vi "Pfeiffer-RVC300.add services.vi"(0 "i ref in":refnum<vi>, 3 "ms timeout (10000)":i32=10000, 5 "error in (no error)":errorcluster) -> (14 "i ref out":refnum<vi>, 17 "timed out":bool, 19 "error out":errorcluster)   [LabVIEW 2014, in "Pfeiffer-RVC300.lvlib"]
doc: "Declares the required DIM services."
uses:
  Pfeiffer-RVC300.lvlib
  Pfeiffer-RVC300.regulation mode.ctl
  CSlibraries-extern/DimLVEvent/LVDimInterface/LVDimInterface.lvlib
  CSCore/CSSystem/CSSystemLib/CSSystemLib.lvlib
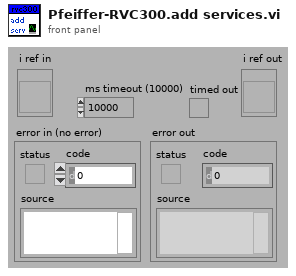
[diagram p1: front panel]
types:
  T1 = typedef "Pfeiffer-RVC300.lvlib/Pfeiffer-RVC300.i attribute.ctl" = cluster{"interfaceInitialized":bool, "VISAResource":refnum<visa-resource-name>, "WaitingTime":u32, "nomValues":T2, "actValues":T2}
  T2 = typedef "Pfeiffer-RVC300.lvlib/Pfeiffer-RVC300.parameters.ctl" = cluster{"regulationMode":T3, "valveType":string, "sensorType":string, "valveState":string, "flow":dbl, "pressure":dbl, "serviceIDs":cluster{"regulationModeID":i32, "valveTypeID":i32, "sensorTypeID":i32, "valveStateID":i32, "flowID":i32, "pressureID":i32}}
  T3 = typedef "Pfeiffer-RVC300.lvlib/Pfeiffer-RVC300.regulation mode.ctl" = enum16{"unknown", "Pressure", "Flow", "Wait"}
  T4 = cluster{"my_serviceID":i32, "my_serviceID":i32, "my_serviceID":i32, "my_serviceID":i32, "my_serviceID":i32, "my_serviceID":i32}
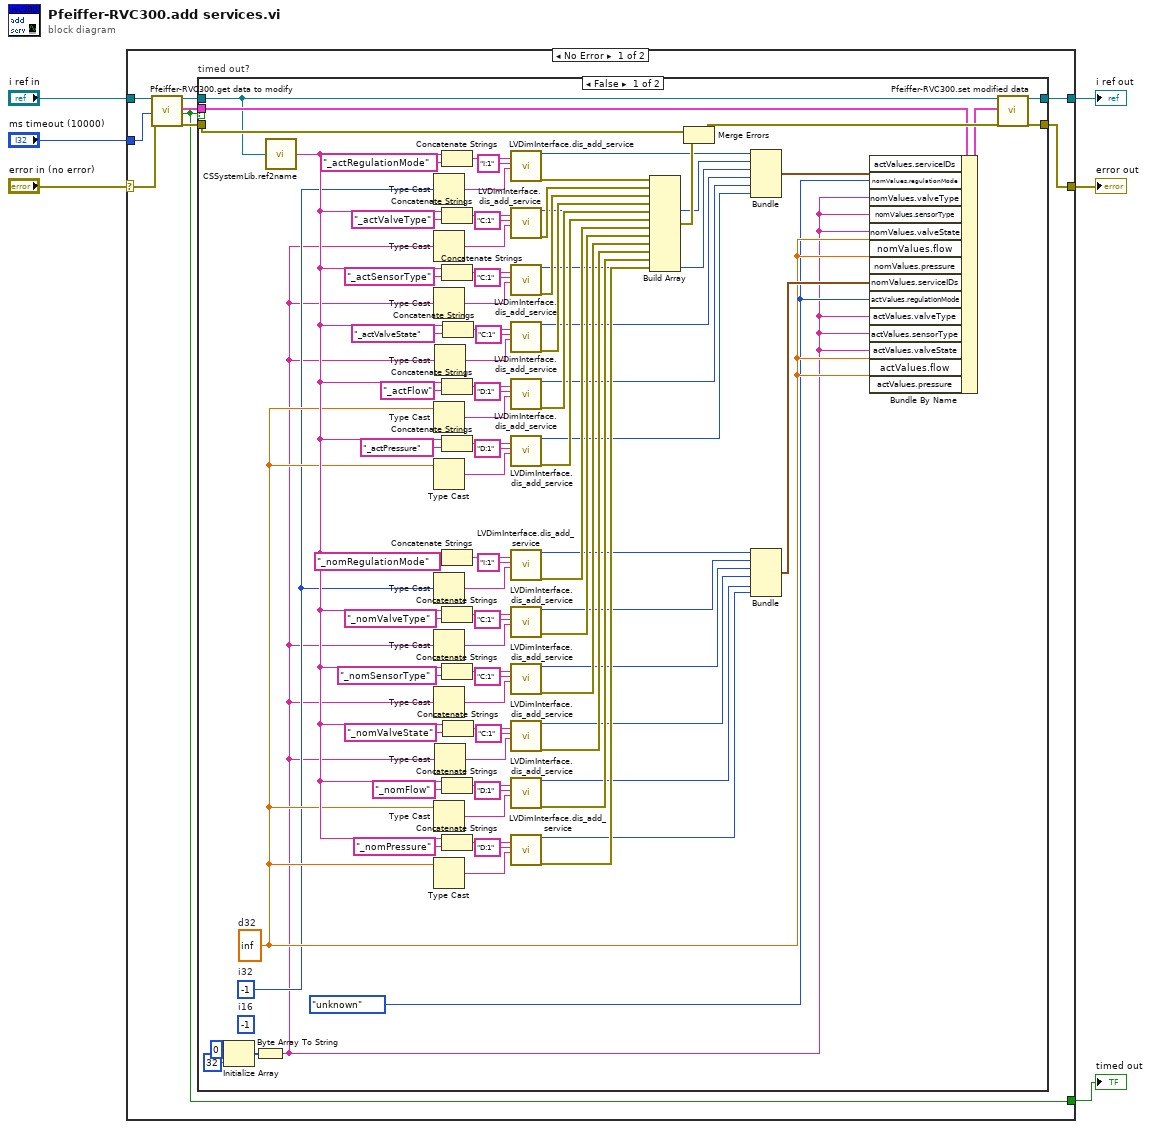
[diagram p0: block diagram]
diagram:
  n1 = case shown="No Error" "error in (no error)" {
    selector: "error in (no error)" -> [w13 w109]
    tunnel: [w9 w109] -> w5
    tunnel: "i ref in" -> [w15 w108]
    tunnel: [w11 w108] -> w3
    tunnel: "ms timeout (10000)" -> [w14 _]
    tunnel: [w8 _] -> w1
    frame No Error {
      n2 = call "Pfeiffer-RVC300.get data to modify.vi"("i ref in"=w15, "ms timeout (10000)"=w14, "error in (no error)"=w13) -> ("i ref out"=w12:refnum<vi>, "i attribute"=w7:T1, "timed out"=w8:bool, "error out"=w10:errorcluster)  [unwired: 13 in]
      n3 = case "timed out?" shown="False" w8 {
        tunnel: w12 -> [w25 w107]
        tunnel: [w105 w107] -> w11
        tunnel: w10 -> [w42 w106]
        tunnel: [w104 w106] -> w9
        tunnel: w7 -> [w39 _]
        frame False {
          w20 = Pfeiffer-RVC300.regulation_mode."unknown" ("actValues.regulationMode")
          (unwired) i16 -1  # i16
          w22 = inf  # d32
          w21 = -1  # i32
          n4 = Initialize Array(u8 0, 32 ("dimension size")) -> (w19:u8[])
          n5 = Byte Array To String(unsigned byte array=w19) -> (string=w16:string)
          n6 = call "CSSystemLib.ref2name.vi"("obj refnum"=w25) -> ("name"=w55:string)
          n7 = Type Cast(x=w21) -> (*(type *) &x=w100:string)  [unwired: 1 in]
          n8 = Type Cast(x=w16) -> (*(type *) &x=w99:string)  [unwired: 1 in]
          n9 = Type Cast(x=w16) -> (*(type *) &x=w92:string)  [unwired: 1 in]
          n10 = Type Cast(x=w22) -> (*(type *) &x=w84:string)  [unwired: 1 in]
          n11 = Type Cast(x=w22) -> (*(type *) &x=w80:string)  [unwired: 1 in]
          n12 = Type Cast(x=w21) -> (*(type *) &x=w76:string)  [unwired: 1 in]
          n13 = Type Cast(x=w16) -> (*(type *) &x=w75:string)  [unwired: 1 in]
          n14 = Type Cast(x=w16) -> (*(type *) &x=w68:string)  [unwired: 1 in]
          n15 = Type Cast(x=w22) -> (*(type *) &x=w60:string)  [unwired: 1 in]
          n16 = Type Cast(x=w22) -> (*(type *) &x=w56:string)  [unwired: 1 in]
          n17 = Type Cast(x=w16) -> (*(type *) &x=w88:string)  [unwired: 1 in]
          n18 = Type Cast(x=w16) -> (*(type *) &x=w64:string)  [unwired: 1 in]
          n19 = Concatenate Strings(w55, "_actRegulationMode" ("string")) -> (w103:string)
          n20 = Concatenate Strings(w55, "_actValveType" ("string")) -> (w96:string)
          n21 = Concatenate Strings(w55, "_actSensorType" ("string")) -> (w95:string)
          n22 = Concatenate Strings(w55, "_actFlow" ("string")) -> (w87:string)
          n23 = Concatenate Strings(w55, "_actPressure" ("string")) -> (w83:string)
          n24 = Concatenate Strings(w55, "_nomRegulationMode" ("string")) -> (w79:string)
          n25 = Concatenate Strings(w55, "_nomValveType" ("string")) -> (w72:string)
          n26 = Concatenate Strings(w55, "_nomSensorType" ("string")) -> (w71:string)
          n27 = Concatenate Strings(w55, "_nomFlow" ("string")) -> (w63:string)
          n28 = Concatenate Strings(w55, "_nomPressure" ("string")) -> (w59:string)
          n29 = Concatenate Strings(w55, "_actValveState" ("string")) -> (w91:string)
          n30 = Concatenate Strings(w55, "_nomValveState" ("string")) -> (w67:string)
          n31 = call "LVDimInterface.dis_add_service.vi"("serviceName"=w103, "typeDescriptor"="I:1", "data"=w100) -> ("my_serviceID"=w38:i32, "error out"=w54:errorcluster)  [unwired: 15 in]
          n32 = call "LVDimInterface.dis_add_service.vi"("serviceName"=w96, "typeDescriptor"="C:1", "data"=w99) -> ("my_serviceID"=w37:i32, "error out"=w53:errorcluster)  [unwired: 15 in]
          n33 = call "LVDimInterface.dis_add_service.vi"("serviceName"=w95, "typeDescriptor"="C:1", "data"=w92) -> ("my_serviceID"=w36:i32, "error out"=w52:errorcluster)  [unwired: 15 in]
          n34 = call "LVDimInterface.dis_add_service.vi"("serviceName"=w91, "typeDescriptor"="C:1", "data"=w88) -> ("my_serviceID"=w35:i32, "error out"=w51:errorcluster)  [unwired: 15 in]
          n35 = call "LVDimInterface.dis_add_service.vi"("serviceName"=w87, "typeDescriptor"="D:1", "data"=w84) -> ("my_serviceID"=w34:i32, "error out"=w50:errorcluster)  [unwired: 15 in]
          n36 = call "LVDimInterface.dis_add_service.vi"("serviceName"=w83, "typeDescriptor"="D:1", "data"=w80) -> ("my_serviceID"=w33:i32, "error out"=w49:errorcluster)  [unwired: 15 in]
          n37 = call "LVDimInterface.dis_add_service.vi"("serviceName"=w79, "typeDescriptor"="I:1", "data"=w76) -> ("my_serviceID"=w32:i32, "error out"=w48:errorcluster)  [unwired: 15 in]
          n38 = call "LVDimInterface.dis_add_service.vi"("serviceName"=w72, "typeDescriptor"="C:1", "data"=w75) -> ("my_serviceID"=w31:i32, "error out"=w47:errorcluster)  [unwired: 15 in]
          n39 = call "LVDimInterface.dis_add_service.vi"("serviceName"=w71, "typeDescriptor"="C:1", "data"=w68) -> ("my_serviceID"=w30:i32, "error out"=w46:errorcluster)  [unwired: 15 in]
          n40 = call "LVDimInterface.dis_add_service.vi"("serviceName"=w67, "typeDescriptor"="C:1", "data"=w64) -> ("my_serviceID"=w29:i32, "error out"=w45:errorcluster)  [unwired: 15 in]
          n41 = call "LVDimInterface.dis_add_service.vi"("serviceName"=w63, "typeDescriptor"="D:1", "data"=w60) -> ("my_serviceID"=w28:i32, "error out"=w44:errorcluster)  [unwired: 15 in]
          n42 = call "LVDimInterface.dis_add_service.vi"("serviceName"=w59, "typeDescriptor"="D:1", "data"=w56) -> ("my_serviceID"=w27:i32, "error out"=w43:errorcluster)  [unwired: 15 in]
          n43 = Build Array(w54, w53, w52, w51, w50, w49, w48, w47, w46, w45, w44, w43) -> (w41:errorcluster[])
          n44 = Merge Errors(w42, w41) -> (w40:errorcluster)
          n45 = Bundle("my_serviceID"=w38, "my_serviceID"=w37, "my_serviceID"=w36, "my_serviceID"=w35, "my_serviceID"=w34, "my_serviceID"=w33) -> (w23:T4)  [unwired: 1 in]
          n46 = Bundle("my_serviceID"=w32, "my_serviceID"=w31, "my_serviceID"=w30, "my_serviceID"=w29, "my_serviceID"=w28, "my_serviceID"=w27) -> (w24:T4)  [unwired: 1 in]
          n47 = Bundle By Name(cluster=w39, "actValues.serviceIDs"=w23, "nomValues.regulationMode"=w20, "nomValues.valveType"=w16, "nomValues.sensorType"=w16, "nomValues.valveState"=w16, "nomValues.flow"=w22, "nomValues.pressure"=w22, "nomValues.serviceIDs"=w24, "actValues.regulationMode"=w20, "actValues.valveType"=w16, "actValues.sensorType"=w16, "actValues.valveState"=w16, "actValues.flow"=w22, "actValues.pressure"=w22) -> (w26:T1)
          n48 = call "Pfeiffer-RVC300.set modified data.vi"("i ref in"=w25, "i attribute"=w26, "error in (no error)"=w40) -> ("i ref out"=w105:refnum<vi>, "error out"=w104:errorcluster)  [unwired: 15 in]
        }
        frame True {
        }
      }
    }
    frame Error {
    }
  }
  "error out" <- w5
  "i ref out" <- w3
  "timed out" <- w1
